vi "sha3_256_string.vi"(11 "Input Text":string) -> (3 "Hash":string)   [LabVIEW 2021]
panel:
  # "Online Calculator\nhttp://emn178.github.io/online-tools/keccak_256.html"
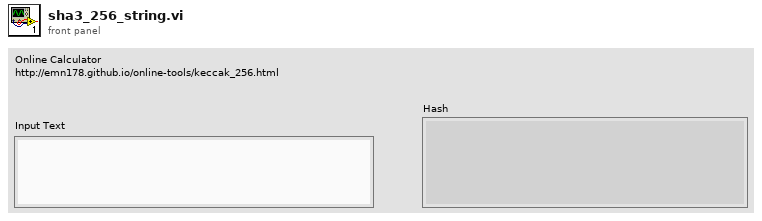
[diagram p1: front panel]
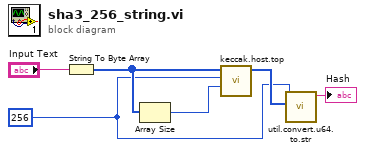
[diagram p0: block diagram]
diagram:
  w1 = 256
  n1 = String To Byte Array(string="Input Text") -> (unsigned byte array=w5:u8[])
  n2 = Array Size(array=w5) -> (size(s)=w4:i32)
  n3 = call "keccak.host.top.vi"("size"=w4, "Bits.in"=w1, "Data.in"=w5) -> ("Final.State"=w3:u64[])  [unwired: 8 in]
  n4 = call "util.convert.u64.to.str.vi"("Final.State"=w3, "Numeric"=w1) -> ("String"=→"Hash":string)  [unwired: 9 in]
